vi "requestNewUserOutputs.vi"(8 "error in (no error)":errorcluster, 11 "Model in":refnum<class "Model.lvclass">) -> (0 "error out":errorcluster, 3 "Model out":refnum<class "Model.lvclass">)   [LabVIEW 2013, in "Model.lvclass"]
uses:
  Model.lvclass
  Model.lvclass/Model.ctl
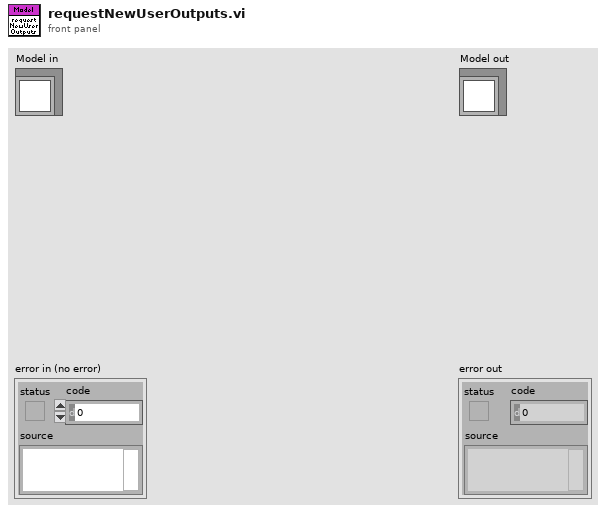
[diagram p1: front panel]
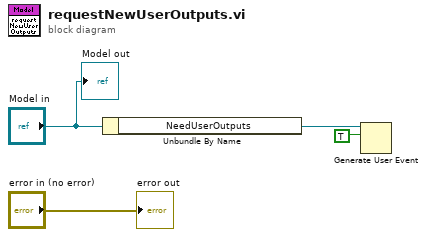
[diagram p0: block diagram]
diagram:
  n1 = Unbundle By Name("Model in") -> ("NeedUserOutputs"=w2:refnum<user-event>)
  n2 = Generate User Event(user event=w2, event data cluster=TRUE) -> ()  [unwired: 2 in, 2 out]
  "error out" <- "error in (no error)"
  "Model out" <- "Model in"
